vi "nanocal -- nuclear schottky fit V7.vi"() -> ()   [LabVIEW 2021] (continued)
 0.022752418474   ,  \"T\" -> 1.130000000000   ,  \"B\" -> 12.000000000000   ,  \"θ\" -> 45.000000000000   ,  \"Reoff\" -> 0.000000000000   ,  \"Imoff\" -> 0.000000000000   ,  \"στ1\" -> 0.000000000000   ,  \"στS\" -> 0.000000000000   ,  \"στN\" -> 0.000000000000    |>   , \r\"IDS0322_210901_RAW_cal__ref_\" ->   <|    \"ζ\" -> 0.019557893298   ,  \"τ1\" -> 0.012446212333   ,  \"τS\" -> 0.011139553358   ,  \"τN\" -> 0.000114229396   ,  \"τC\" -> 0.005115315079   ,  \"κ0\" -> 0.000000013115   ,  \"mm1\" -> 0.000067933462   ,  \"mm2\" -> 0.012117833487   ,  \"mm3\" -> 0.016849643499   ,  \"T\" -> 1.900000000000   ,  \"B\" -> 12.000000000000   ,  \"θ\" -> 45.000000000000   ,  \"Reoff\" -> 0.000000000000   ,  \"Imoff\" -> 0.000000000000   ,  \"στ1\" -> 0.000000000000   ,  \"στS\" -> 0.000000000000   ,  \"στN\" -> 0.000000000000    |>   , \r\"IDS0322_210901_RAW_cal__sam_\" ->   <|    \"ζ\" -> 0.018090572724   ,  \"τ1\" -> 0.013314780956   ,  \"τS\" -> 0.010820835010   ,  \"τN\" -> 0.000265552167   ,  \"τC\" -> 0.005393540417   ,  \"κ0\" -> 0.000000013100   ,  \"mm1\" -> 0.000064590824   ,  \"mm2\" -> 0.012452255889   ,  \"mm3\" -> 0.017478420931   ,  \"T\" -> 1.900000000000   ,  \"B\" -> 12.000000000000   ,  \"θ\" -> 45.000000000000   ,  \"Reoff\" -> 0.000000000000   ,  \"Imoff\" -> 0.000000000000   ,  \"στ1\" -> 0.000000000000   ,  \"στS\" -> 0.000000000000   ,  \"στN\" -> 0.000000000000    |>   , \r\"IDS0323_210901_RAW_cal__ref_\" ->   <|    \"ζ\" -> 0.018290634783   ,  \"τ1\" -> 0.011707989393   ,  \"τS\" -> 0.007391181448   ,  \"τN\" -> 0.000042685582   ,  \"τC\" -> 0.004638632451   ,  \"κ0\" -> 0.000000023525   ,  \"mm1\" -> 0.000051768819   ,  \"mm2\" -> 0.011185443963   ,  \"mm3\" -> 0.012679246238   ,  \"T\" -> 3.100000000000   ,  \"B\" -> 12.000000000000   ,  \"θ\" -> 45.000000000000   ,  \"Reoff\" -> 0.000000000000   ,  \"Imoff\" -> 0.000000000000   ,  \"στ1\" -> 0.000000000000   ,  \"στS\" -> 0.000000000000   ,  \"στN\" -> 0.000000000000    |>   , \r\"IDS0323_210901_RAW_cal__sam_\" ->   <|    \"ζ\" -> 0.019438138135   ,  \"τ1\" -> 0.013521019406   ,  \"τS\" -> 0.007253169401   ,  \"τN\" -> 0.000154824830   ,  \"τC\" -> 0.004746579385   ,  \"κ0\" -> 0.000000023466   ,  \"mm1\" -> 0.000055371802   ,  \"mm2\" -> 0.011289401344   ,  \"mm3\" -> 0.014474817491   ,  \"T\" -> 3.100000000000   ,  \"B\" -> 12.000000000000   ,  \"θ\" -> 45.000000000000   ,  \"Reoff\" -> 0.000000000000   ,  \"Imoff\" -> 0.000000000000   ,  \"στ1\" -> 0.000000000000   ,  \"στS\" -> 0.000000000000   ,  \"στN\" -> 0.000000000000    |>   , \r\"IDS0324_210901_RAW_cal__ref_\" ->   <|    \"ζ\" -> 0.016342153608   ,  \"τ1\" -> 0.012470308436   ,  \"τS\" -> 0.004793459347   ,  \"τN\" -> 0.000012881713   ,  \"τC\" -> 0.003213848745   ,  \"κ0\" -> 0.000000058321   ,  \"mm1\" -> 0.000031257206   ,  \"mm2\" -> 0.008030763960   ,  \"mm3\" -> 0.012507023039   ,  \"T\" -> 5.700000000000   ,  \"B\" -> 12.000000000000   ,  \"θ\" -> 45.000000000000   ,  \"Reoff\" -> 0.000000000000   ,  \"Imoff\" -> 0.000000000000   ,  \"στ1\" -> 0.000000000000   ,  \"στS\" -> 0.000000000000   ,  \"στN\" -> 0.000000000000    |>   , \r\"IDS0324_210901_RAW_cal__sam_\" ->   <|    \"ζ\" -> 0.018573189054   ,  \"τ1\" -> 0.013304612245   ,  \"τS\" -> 0.003723860844   ,  \"τN\" -> 0.000084829442   ,  \"τC\" -> 0.004309703632   ,  \"κ0\" -> 0.000000058362   ,  \"mm1\" -> 0.000036954445   ,  \"mm2\" -> 0.007938616076   ,  \"mm3\" -> 0.013518175167   ,  \"T\" -> 5.700000000000   ,  \"B\" -> 12.000000000000   ,  \"θ\" -> 45.000000000000   ,  \"Reoff\" -> 0.000000000000   ,  \"Imoff\" -> 0.000000000000   ,  \"στ1\" -> 0.000000000000   ,  \"στS\" -> 0.000000000000   ,  \"στN\" -> 0.000000000000    |>   , \r\"IDS0330_210901_RAW_cal__ref_\" ->   <|    \"ζ\" -> 0.000000000000   ,  \"τ1\" -> 0.000000000000   ,  \"τS\" -> 0.000000000000   ,  \"τN\" -> 0.000000000000   ,  \"τC\" -> 0.000000000000   ,  \"κ0\" -> 0.000000000000   ,  \"mm1\" -> 0.000000000000   ,  \"mm2\" -> 0.000000000000   ,  \"mm3\" -> 0.000000000000   ,  \"T\" -> 0.197000000000   ,  \"B\" -> 1.000000000000   ,  \"θ\" -> 90.000000000000   ,  \"Reoff\" -> 0.000000000000   ,  \"Imoff\" -> 0.000000000000   ,  \"στ1\" -> 0.000000000000   ,  \"στS\" -> 0.000000000000   ,  \"στN\" -> 0.000000000000    |>   , \r\"IDS0330_210901_RAW_cal__sam_\" ->   <|    \"ζ\" -> 0.000000000000   ,  \"τ1\" -> 0.000000000000   ,  \"τS\" -> 0.000000000000   ,  \"τN\" -> 0.000000000000   ,  \"τC\" -> 0.000000000000   ,  \"κ0\" -> 0.000000000000   ,  \"mm1\" -> 0.000000000000   ,  \"mm2\" -> 0.000000000000   ,  \"mm3\" -> 0.000000000000   ,  \"T\" -> 0.197000000000   ,  \"B\" -> 1.000000000000   ,  \"θ\" -> 90.000000000000   ,  \"Reoff\" -> 0.000000000000   ,  \"Imoff\" -> 0.000000000000   ,  \"στ1\" -> 0.000000000000   ,  \"στS\" -> 0.000000000000   ,  \"στN\" -> 0.000000000000    |>   , \r\"IDS0331_210901_RAW_cal__ref_\" ->   <|    \"ζ\" -> 0.000000000000   ,  \"τ1\" -> 0.000000000000   ,  \"τS\" -> 0.000000000000   ,  \"τN\" -> 0.000000000000   ,  \"τC\" -> 0.000000000000   ,  \"κ0\" -> 0.000000000000   ,  \"mm1\" -> 0.000000000000   ,  \"mm2\" -> 0.000000000000   ,  \"mm3\" -> 0.000000000000   ,  \"T\" -> 0.197000000000   ,  \"B\" -> 2.000000000000   ,  \"θ\" -> 90.000000000000   ,  \"Reoff\" -> 0.000000000000   ,  \"Imoff\" -> 0.000000000000   ,  \"στ1\" -> 0.000000000000   ,  \"στS\" -> 0.000000000000   ,  \"στN\" -> 0.000000000000    |>   , \r\"IDS0331_210901_RAW_cal__sam_\" ->   <|    \"ζ\" -> 0.000000000000   ,  \"τ1\" -> 0.000000000000   ,  \"τS\" -> 0.000000000000   ,  \"τN\" -> 0.000000000000   ,  \"τC\" -> 0.000000000000   ,  \"κ0\" -> 0.000000000000   ,  \"mm1\" -> 0.000000000000   ,  \"mm2\" -> 0.000000000000   ,  \"mm3\" -> 0.000000000000   ,  \"T\" -> 0.197000000000   ,  \"B\" -> 2.000000000000   ,  \"θ\" -> 90.000000000000   ,  \"Reoff\" -> 0.000000000000   ,  \"Imoff\" -> 0.000000000000   ,  \"στ1\" -> 0.000000000000   ,  \"στS\" -> 0.000000000000   ,  \"στN\" -> 0.000000000000    |>   , \r\"IDS0335_210904_RAW_cal__ref_\" ->   <|    \"ζ\" -> 0.206204028371   ,  \"τ1\" -> 0.030267809159   ,  \"τS\" -> 0.083699658284   ,  \"τN\" -> 0.011315524001   ,  \"τC\" -> 0.001118356963   ,  \"κ0\" -> 0.000000001029   ,  \"mm1\" -> 0.000189441796   ,  \"mm2\" -> 0.025670987536   ,  \"mm3\" -> 0.120133432419   ,  \"T\" -> 0.197000000000   ,  \"B\" -> 5.000000000000   ,  \"θ\" -> 90.000000000000   ,  \"Reoff\" -> -27794554.455445542900   ,  \"Imoff\" -> 0.000000000000   ,  \"στ1\" -> 0.030199688034   ,  \"στS\" -> 0.003526382549   ,  \"στN\" -> 0.000000000000    |>   , \r\"IDS0335_210904_RAW_cal__sam_\" ->   <|    \"ζ\" -> 0.127476550533   ,  \"τ1\" -> 0.026692349363   ,  \"τS\" -> 0.111739634553   ,  \"τN\" -> 0.012149249884   ,  \"τC\" -> 0.001469649387   ,  \"κ0\" -> 0.000000001130   ,  \"mm1\" -> 0.000164458900   ,  \"mm2\" -> 0.023578369229   ,  \"mm3\" -> 0.144100982695   ,  \"T\" -> 0.197000000000   ,  \"B\" -> 5.000000000000   ,  \"θ\" -> 90.000000000000   ,  \"Reoff\" -> -19117469.879518091700   ,  \"Imoff\" -> 0.000000000000   ,  \"στ1\" -> 0.000000000000   ,  \"στS\" -> 0.000000000000   ,  \"στN\" -> 0.000000000000    |>   , \r\"IDS0336_210904_RAW_cal__ref_\" ->   <|    \"ζ\" -> 0.369061948092   ,  \"τ1\" -> 0.041711176697   ,  \"τS\" -> 0.225950048302   ,  \"τN\" -> 0.066003099748   ,  \"τC\" -> 0.001407606072   ,  \"κ0\" -> 0.000000000381   ,  \"mm1\" -> 0.000378190489   ,  \"mm2\" -> 0.031503380077   ,  \"mm3\" -> 0.410939157824   ,  \"T\" -> 0.122000000000   ,  \"B\" -> 5.000000000000   ,  \"θ\" -> 90.000000000000   ,  \"Reoff\" -> -46126237.623762376600   ,  \"Imoff\" -> 0.000000000000   ,  \"στ1\" -> 0.041981174011   ,  \"στS\" -> 0.019738908124   ,  \"στN\" -> 0.000000000000    |>   , \r\"IDS0336_210904_RAW_cal__sam_\" ->   <|    \"ζ\" -> 0.192483765517   ,  \"τ1\" -> 0.038218926206   ,  \"τS\" -> 0.302700165376   ,  \"τN\" -> 0.092288910100   ,  \"τC\" -> 0.001788727736   ,  \"κ0\" -> 0.000000000500   ,  \"mm1\" -> 0.000287527431   ,  \"mm2\" -> 0.028741269140   ,  \"mm3\" -> 0.481996917433   ,  \"T\" -> 0.122000000000   ,  \"B\" -> 5.000000000000   ,  \"θ\" -> 90.000000000000   ,  \"Reoff\" -> 0.000000000000   ,  \"Imoff\" -> 0.000000000000   ,  \"στ1\" -> 0.000000000000   ,  \"στS\" -> 0.000000000000   ,  \"στN\" -> 0.000000000000    |>   , \r\"IDS0337_210904_RAW_cal__ref_\" ->   <|    \"ζ\" -> 0.291494561804   ,  \"τ1\" -> 0.036667876547   ,  \"τS\" -> 0.128215599927   ,  \"τN\" -> 0.021540574973   ,  \"τC\" -> 0.001127155281   ,  \"κ0\" -> 0.000000000640   ,  \"mm1\" -> 0.000253065243   ,  \"mm2\" -> 0.030442060863   ,  \"mm3\" -> 0.200509191202   ,  \"T\" -> 0.157000000000   ,  \"B\" -> 5.000000000000   ,  \"θ\" -> 90.000000000000   ,  \"Reoff\" -> -62465346.534653462500   ,  \"Imoff\" -> 0.000000000000   ,  \"στ1\" -> 0.039211636627   ,  \"στS\" -> 0.006414125500   ,  \"στN\" -> 0.000000000000    |>   , \r\"IDS0337_210904_RAW_cal__sam_\" ->   <|    \"ζ\" -> 0.174989526301   ,  \"τ1\" -> 0.032277116931   ,  \"τS\" -> 0.156061636315   ,  \"τN\" -> 0.033861256896   ,  \"τC\" -> 0.001461638306   ,  \"κ0\" -> 0.000000000742   ,  \"mm1\" -> 0.000216209109   ,  \"mm2\" -> 0.025810900049   ,  \"mm3\" -> 0.230869056407   ,  \"T\" -> 0.157000000000   ,  \"B\" -> 5.000000000000   ,  \"θ\" -> 90.000000000000   ,  \"Reoff\" -> -41753012.048192769300   ,  \"Imoff\" -> 0.000000000000   ,  \"στ1\" -> 0.000000000000   ,  \"στS\" -> 0.000000000000   ,  \"στN\" -> 0.000000000000    |>   , \r\"IDS0338_210904_RAW_cal__ref_\" ->   <|    \"ζ\" -> 0.269633076560   ,  \"τ1\" -> 0.032794135380   ,  \"τS\" -> 0.108453011647   ,  \"τN\" -> 0.017260666597   ,  \"τC\" -> 0.001066919164   ,  \"κ0\" -> 0.000000000733   ,  \"mm1\" -> 0.000225204386   ,  \"mm2\" -> 0.027393186252   ,  \"mm3\" -> 0.165852907980   ,  \"T\" -> 0.170000000000   ,  \"B\" -> 5.000000000000   ,  \"θ\" -> 90.000000000000   ,  \"Reoff\" -> -53299504.950495049400   ,  \"Imoff\" -> 0.000000000000   ,  \"στ1\" -> 0.032867428442   ,  \"στS\" -> 0.004982833917   ,  \"στN\" -> 0.000000000000    |>   , \r\"IDS0338_210904_RAW_cal__sam_\" ->   <|    \"ζ\" -> 0.165649151389   ,  \"τ1\" -> 0.028874600848   ,  \"τS\" -> 0.141983523605   ,  \"τN\" -> 0.021766467668   ,  \"τC\" -> 0.001383503895   ,  \"κ0\" -> 0.000000000838   ,  \"mm1\" -> 0.000195205233   ,  \"mm2\" -> 0.024502619119   ,  \"mm3\" -> 0.196435318758   ,  \"T\" -> 0.170000000000   ,  \"B\" -> 5.000000000000   ,  \"θ\" -> 90.000000000000   ,  \"Reoff\" -> -35397590.361445784600   ,  \"Imoff\" -> 0.000000000000   ,  \"στ1\" -> 0.000000000000   ,  \"στS\" -> 0.000000000000   ,  \"στN\" -> 0.000000000000    |>   , \r\"IDS0339_210904_RAW_cal__ref_\" ->   <|    \"ζ\" -> 0.118223949911   ,  \"τ1\" -> 0.026953810816   ,  \"τS\" -> 0.059687464570   ,  \"τN\" -> 0.005813068847   ,  \"τC\" -> 0.001318135171   ,  \"κ0\" -> 0.000000001341   ,  \"mm1\" -> 0.000136934905   ,  \"mm2\" -> 0.023512775569   ,  \"mm3\" -> 0.077866500712   ,  \"T\" -> 0.255000000000   ,  \"B\" -> 5.000000000000   ,  \"θ\" -> 90.000000000000   ,  \"Reoff\" -> -14245049.504950493600   ,  \"Imoff\" -> 0.000000000000   ,  \"στ1\" -> 0.036632926849   ,  \"στS\" -> 0.002605706336   ,  \"στN\" -> 0.000000000000    |>   , \r\"IDS0339_210904_RAW_cal__sam_\" ->   <|    \"ζ\" -> 0.070510248751   ,  \"τ1\" -> 0.022152847239   ,  \"τS\" -> 0.078660981887   ,  \"τN\" -> 0.006346817462   ,  \"τC\" -> 0.001852903257   ,  \"κ0\" -> 0.000000001477   ,  \"mm1\" -> 0.000119580835   ,  \"mm2\" -> 0.020081415868   ,  \"mm3\" -> 0.094806474219   ,  \"T\" -> 0.255000000000   ,  \"B\" -> 5.000000000000   ,  \"θ\" -> 90.000000000000   ,  \"Reoff\" -> -9000000.000000000000   ,  \"Imoff\" -> 0.000000000000   ,  \"στ1\" -> 0.000000000000   ,  \"στS\" -> 0.000000000000   ,  \"στN\" -> 0.000000000000    |>   , \r\"IDS0340_210904_RAW_cal__ref_\" ->   <|    \"ζ\" -> 0.082410022210   ,  \"τ1\" -> 0.025302969896   ,  \"τS\" -> 0.049616733190   ,  \"τN\" -> 0.002823484973   ,  \"τC\" -> 0.001541432070   ,  \"κ0\" -> 0.000000001718   ,  \"mm1\" -> 0.000114319399   ,  \"mm2\" -> 0.023099438171   ,  \"mm3\" -> 0.060392462102   ,  \"T\" -> 0.308000000000   ,  \"B\" -> 5.000000000000   ,  \"θ\" -> 90.000000000000   ,  \"Reoff\" -> -7868811.881188109520   ,  \"Imoff\" -> 0.000000000000   ,  \"στ1\" -> 0.036552733909   ,  \"στS\" -> 0.001615668069   ,  \"στN\" -> 0.000000000000    |>   , \r\"IDS0340_210904_RAW_cal__sam_\" ->   <|    \"ζ\" -> 0.049192434897   ,  \"τ1\" -> 0.021139048522   ,  \"τS\" -> 0.064524263818   ,  \"τN\" -> 0.003413094239   ,  \"τC\" -> 0.002227810965   ,  \"κ0\" -> 0.000000001879   ,  \"mm1\" -> 0.000101271202   ,  \"mm2\" -> 0.019728994700   ,  \"mm3\" -> 0.074815955705   ,  \"T\" -> 0.308000000000   ,  \"B\" -> 5.000000000000   ,  \"θ\" -> 90.000000000000   ,  \"Reoff\" -> -4933734.939759036530   ,  \"Imoff\" -> 0.000000000000   ,  \"στ1\" -> 0.000000000000   ,  \"στS\" -> 0.000000000000   ,  \"στN\" -> 0.000000000000    |>   , \r\"IDS0341_210904_RAW_cal__ref_\" ->   <|    \"ζ\" -> 0.059535652055   ,  \"τ1\" -> 0.024399428177   ,  \"τS\" -> 0.042628676419   ,  \"τN\" -> 0.001866665396   ,  \"τC\" -> 0.001976492813   ,  \"κ0\" -> 0.000000002092   ,  \"mm1\" -> 0.000106643977   ,  \"mm2\" -> 0.022574580065   ,  \"mm3\" -> 0.050839097951   ,  \"T\" -> 0.360000000000   ,  \"B\" -> 5.000000000000   ,  \"θ\" -> 90.000000000000   ,  \"Reoff\" -> -3485148.514851480720   ,  \"Imoff\" -> 0.000000000000   ,  \"στ1\" -> 0.049517186258   ,  \"στS\" -> 0.001491570893   ,  \"στN\" -> 0.000000000000    |>   , \r\"IDS0341_210904_RAW_cal__sam_\" ->   <|    \"ζ\" -> 0.036062522071   ,  \"τ1\" -> 0.018116162768   ,  \"τS\" -> 0.055032833309   ,  \"τN\" -> 0.002026723445   ,  \"τC\" -> 0.002755523522   ,  \"κ0\" -> 0.000000002282   ,  \"mm1\" -> 0.000091630452   ,  \"mm2\" -> 0.017261892165   ,  \"mm3\" -> 0.062635431951   ,  \"T\" -> 0.360000000000   ,  \"B\" -> 5.000000000000   ,  \"θ\" -> 90.000000000000   ,  \"Reoff\" -> -2587349.397590361540   ,  \"Imoff\" -> 0.000000000000   ,  \"στ1\" -> 0.000000000000   ,  \"στS\" -> 0.000000000000   ,  \"στN\" -> 0.000000000000    |>   , \r\"IDS0342_210904_RAW_cal__ref_\" ->   <|    \"ζ\" -> 0.044694741546   ,  \"τ1\" -> 0.020073823055   ,  \"τS\" -> 0.035925122531   ,  \"τN\" -> 0.001180968193   ,  \"τC\" -> 0.002238294537   ,  \"κ0\" -> 0.000000002627   ,  \"mm1\" -> 0.000090575996   ,  \"mm2\" -> 0.018946622284   ,  \"mm3\" -> 0.042039457171   ,  \"T\" -> 0.438000000000   ,  \"B\" -> 5.000000000000   ,  \"θ\" -> 90.000000000000   ,  \"Reoff\" -> -2688118.811881184580   ,  \"Imoff\" -> 0.000000000000   ,  \"στ1\" -> 0.000000000000   ,  \"στS\" -> 0.000039598396   ,  \"στN\" -> 0.000000000000    |>   , \r\"IDS0342_210904_RAW_cal__sam_\" ->   <|    \"ζ\" -> 0.027534849374   ,  \"τ1\" -> 0.019066527741   ,  \"τS\" -> 0.046236587360   ,  \"τN\" -> 0.001227722560   ,  \"τC\" -> 0.003332461518   ,  \"κ0\" -> 0.000000002852   ,  \"mm1\" -> 0.000083583563   ,  \"mm2\" -> 0.018352322518   ,  \"mm3\" -> 0.052734315722   ,  \"T\" -> 0.438000000000   ,  \"B\" -> 5.000000000000   ,  \"θ\" -> 90.000000000000   ,  \"Reoff\" -> -1846385.542168676850   ,  \"Imoff\" -> 0.000000000000   ,  \"στ1\" -> 0.000000000000   ,  \"στS\" -> 0.000000000000   ,  \"στN\" -> 0.000000000000    |>   , \r\"IDS0343_210904_RAW_cal__ref_\" ->   <|    \"ζ\" -> 0.035816355504   ,  \"τ1\" -> 0.018852618665   ,  \"τS\" -> 0.030539930714   ,  \"τN\" -> 0.000576682499   ,  \"τC\" -> 0.002754969701   ,  \"κ0\" -> 0.000000003271   ,  \"mm1\" -> 0.000087853298   ,  \"mm2\" -> 0.018179313354   ,  \"mm3\" -> 0.035571518608   ,  \"T\" -> 0.530000000000   ,  \"B\" -> 5.000000000000   ,  \"θ\" -> 90.000000000000   ,  \"Reoff\" -> -1891089.108910888430   ,  \"Imoff\" -> 0.000000000000   ,  \"στ1\" -> 0.000000000000   ,  \"στS\" -> 0.000000000000   ,  \"στN\" -> 0.000000000000    |>   , \r\"IDS0343_210904_RAW_cal__sam_\" ->   <|    \"ζ\" -> 0.023098882919   ,  \"τ1\" -> 0.017709986922   ,  \"τS\" -> 0.038881575014   ,  \"τN\" -> 0.000747654909   ,  \"τC\" -> 0.003803962289   ,  \"κ0\" -> 0.000000003538   ,  \"mm1\" -> 0.000078528513   ,  \"mm2\" -> 0.017209583260   ,  \"mm3\" -> 0.044770458303   ,  \"T\" -> 0.530000000000   ,  \"B\" -> 5.000000000000   ,  \"θ\" -> 90.000000000000   ,  \"Reoff\" -> -1599397.590361446140   ,  \"Imoff\" -> 0.000000000000   ,  \"στ1\" -> 0.000000000000   ,  \"στS\" -> 0.000000000000   ,  \"στN\" -> 0.000000000000    |>   , \r\"IDS0344_210904_RAW_cal__ref_\" ->   <|    \"ζ\" -> 0.030262302634   ,  \"τ1\" -> 0.017398280529   ,  \"τS\" -> 0.027078056707   ,  \"τN\" -> 0.000382363637   ,  \"τC\" -> 0.002680781698   ,  \"κ0\" -> 0.000000003878   ,  \"mm1\" -> 0.000072009464   ,  \"mm2\" -> 0.016908620237   ,  \"mm3\" -> 0.031389868421   ,  \"T\" -> 0.620000000000   ,  \"B\" -> 5.000000000000   ,  \"θ\" -> 90.000000000000   ,  \"Reoff\" -> -1891089.108910888430   ,  \"Imoff\" -> 0.000000000000   ,  \"στ1\" -> 0.000000000000   ,  \"στS\" -> 0.000000000000   ,  \"στN\" -> 0.000000000000    |>   , \r\"IDS0344_210904_RAW_cal__sam_\" ->   <|    \"ζ\" -> 0.019239644947   ,  \"τ1\" -> 0.016162010817   ,  \"τS\" -> 0.033688234899   ,  \"τN\" -> 0.000426792406   ,  \"τC\" -> 0.004393456024   ,  \"κ0\" -> 0.000000004224   ,  \"mm1\" -> 0.000073664779   ,  \"mm2\" -> 0.015859557336   ,  \"mm3\" -> 0.039393633044   ,  \"T\" -> 0.620000000000   ,  \"B\" -> 5.000000000000   ,  \"θ\" -> 90.000000000000   ,  \"Reoff\" -> -1105421.686746988450   ,  \"Imoff\" -> 0.000000000000   ,  \"στ1\" -> 0.000000000000   ,  \"στS\" -> 0.000000000000   ,  \"στN\" -> 0.000000000000    |>   , \r\"IDS0346_210904_RAW_cal__ref_\" ->   <|    \"ζ\" -> 0.358342122070   ,  \"τ1\" -> 0.051761802826   ,  \"τS\" -> 0.089859508524   ,  \"τN\" -> 0.270637714066   ,  \"τC\" -> 0.001160576368   ,  \"κ0\" -> 0.000000000399   ,  \"mm1\" -> 0.000303997839   ,  \"mm2\" -> 0.011999269265   ,  \"mm3\" -> 0.530297674424   ,  \"T\" -> 0.122000000000   ,  \"B\" -> 8.000000000000   ,  \"θ\" -> 90.000000000000   ,  \"Reoff\" -> -78405940.594059407700   ,  \"Imoff\" -> 0.000000000000   ,  \"στ1\" -> 0.018696549634   ,  \"στS\" -> 0.010329197801   ,  \"στN\" -> 0.000000000000    |>   , \r\"IDS0346_210904_RAW_cal__sam_\" ->   <|    \"ζ\" -> 0.199267253863   ,  \"τ1\" -> 0.050205114691   ,  \"τS\" -> 0.125855812683   ,  \"τN\" -> 0.296749666016   ,  \"τC\" -> 0.001624351903   ,  \"κ0\" -> 0.000000000535   ,  \"mm1\" -> 0.000267463038   ,  \"mm2\" -> 0.014047868056   ,  \"mm3\" -> 0.544331047407   ,  \"T\" -> 0.122000000000   ,  \"B\" -> 8.000000000000   ,  \"θ\" -> 90.000000000000   ,  \"Reoff\" -> -35716867.469879508000   ,  \"Imoff\" -> 0.000000000000   ,  \"στ1\" -> 0.000000000000   ,  \"στS\" -> 0.000000000000   ,  \"στN\" -> 0.000000000000    |>   , \r\"IDS0347_210906_RAW_cal__ref_\" ->   <|    \"ζ\" -> 0.284128861979   ,  \"τ1\" -> 0.040855237949   ,  \"τS\" -> 0.067239160062   ,  \"τN\" -> 0.100640688459   ,  \"τC\" -> 0.001094387721   ,  \"κ0\" -> 0.000000000641   ,  \"mm1\" -> 0.000239752131   ,  \"mm2\" -> 0.014685784170   ,  \"mm3\" -> 0.242603448199   ,  \"T\" -> 0.157000000000   ,  \"B\" -> 8.000000000000   ,  \"θ\" -> 90.000000000000   ,  \"Reoff\" -> -67247524.752475246800   ,  \"Imoff\" -> 0.000000000000   ,  \"στ1\" -> 0.009528946219   ,  \"στS\" -> 0.006641775518   ,  \"στN\" -> 0.000000000000    |>   , \r\"IDS0347_210906_RAW_cal__sam_\" ->   <|    \"ζ\" -> 0.169709128246   ,  \"τ1\" -> 0.042569783210   ,  \"τS\" -> 0.096466158196   ,  \"τN\" -> 0.116379310482   ,  \"τC\" -> 0.001498996005   ,  \"κ0\" -> 0.000000000766   ,  \"mm1\" -> 0.000215022431   ,  \"mm2\" -> 0.017656553883   ,  \"mm3\" -> 0.275164490520   ,  \"T\" -> 0.157000000000   ,  \"B\" -> 8.000000000000   ,  \"θ\" -> 90.000000000000   ,  \"Reoff\" -> -35716867.469879508000   ,  \"Imoff\" -> 0.000000000000   ,  \"στ1\" -> 0.000000000000   ,  \"στS\" -> 0.000000000000   ,  \"στN\" -> 0.000000000000    |>   , \r\"IDS0348_210906_RAW_cal__ref_\" ->   <|    \"ζ\" -> 0.229184446116   ,  \"τ1\" -> 0.036521753559   ,  \"τS\" -> 0.056643116422   ,  \"τN\" -> 0.063013769225   ,  \"τC\" -> 0.001114108457   ,  \"κ0\" -> 0.000000000764   ,  \"mm1\" -> 0.000205034245   ,  \"mm2\" -> 0.015217532140   ,  \"mm3\" -> 0.169293678338   ,  \"T\" -> 0.178000000000   ,  \"B\" -> 8.000000000000   ,  \"θ\" -> 90.000000000000   ,  \"Reoff\" -> -44930693.069306924900   ,  \"Imoff\" -> 0.000000000000   ,  \"στ1\" -> 0.007491304915   ,  \"στS\" -> 0.004191211320   ,  \"στN\" -> 0.000000000000    |>   , \r\"IDS0348_210906_RAW_cal__sam_\" ->   <|    \"ζ\" -> 0.135783247929   ,  \"τ1\" -> 0.037121050091   ,  \"τS\" -> 0.079201640502   ,  \"τN\" -> 0.079201640502   ,  \"τC\" -> 0.001474311209   ,  \"κ0\" -> 0.000000000894   ,  \"mm1\" -> 0.000173730712   ,  \"mm2\" -> 0.016810842330   ,  \"mm3\" -> 0.201522581240   ,  \"T\" -> 0.178000000000   ,  \"B\" -> 8.000000000000   ,  \"θ\" -> 90.000000000000   ,  \"Reoff\" -> -29680722.891566276600   ,  \"Imoff\" -> 0.000000000000   ,  \"στ1\" -> 0.000000000000   ,  \"στS\" -> 0.000000000000   ,  \"στN\" -> 0.000000000000    |>   , \r\"IDS0349_210906_RAW_cal__ref_\" ->   <|    \"ζ\" -> 0.190984000958   ,  \"τ1\" -> 0.032898392235   ,  \"τS\" -> 0.053015075726   ,  \"τN\" -> 0.036446539803   ,  \"τC\" -> 0.001170894868   ,  \"κ0\" -> 0.000000001035   ,  \"mm1\" -> 0.000184864342   ,  \"mm2\" -> 0.017107531018   ,  \"mm3\" -> 0.123324244538   ,  \"T\" -> 0.200000000000   ,  \"B\" -> 8.000000000000   ,  \"θ\" -> 90.000000000000   ,  \"Reoff\" -> -24207920.792079202800   ,  \"Imoff\" -> 0.000000000000   ,  \"στ1\" -> 0.007827965999   ,  \"στS\" -> 0.003040573624   ,  \"στN\" -> 0.000000000000    |>   , \r\"IDS0349_210906_RAW_cal__sam_\" ->   <|    \"ζ\" -> 0.113690190882   ,  \"τ1\" -> 0.032691214581   ,  \"τS\" -> 0.068786957350   ,  \"τN\" -> 0.048058332081   ,  \"τC\" -> 0.001613875480   ,  \"κ0\" -> 0.000000001156   ,  \"mm1\" -> 0.000161675745   ,  \"mm2\" -> 0.017372504664   ,  \"mm3\" -> 0.146900362342   ,  \"T\" -> 0.200000000000   ,  \"B\" -> 8.000000000000   ,  \"θ\" -> 90.000000000000   ,  \"Reoff\" -> -14590361.445783138300   ,  \"Imoff\" -> 0.000000000000   ,  \"στ1\" -> 0.000000000000   ,  \"στS\" -> 0.000000000000   ,  \"στN\" -> 0.000000000000    |>   , \r\"IDS0350_210906_RAW_cal__ref_\" ->   <|    \"ζ\" -> 0.117284187691   ,  \"τ1\" -> 0.026970666142   ,  \"τS\" -> 0.042347096729   ,  \"τN\" -> 0.016129848116   ,  \"τC\" -> 0.001330224146   ,  \"κ0\" -> 0.000000001350   ,  \"mm1\" -> 0.000136193348   ,  \"mm2\" -> 0.017132196816   ,  \"mm3\" -> 0.076367865944   ,  \"T\" -> 0.260000000000   ,  \"B\" -> 8.000000000000   ,  \"θ\" -> 90.000000000000   ,  \"Reoff\" -> -13846534.653465345500   ,  \"Imoff\" -> 0.000000000000   ,  \"στ1\" -> 0.008626446357   ,  \"στS\" -> 0.001916708788   ,  \"στN\" -> 0.000000000000    |>   , \r\"IDS0350_210906_RAW_cal__sam_\" ->   <|    \"ζ\" -> 0.071614468485   ,  \"τ1\" -> 0.024327525692   ,  \"τS\" -> 0.055056024171   ,  \"τN\" -> 0.019709093999   ,  \"τC\" -> 0.001754398678   ,  \"κ0\" -> 0.000000001497   ,  \"mm1\" -> 0.000114067222   ,  \"mm2\" -> 0.016460052715   ,  \"mm3\" -> 0.089627186802   ,  \"T\" -> 0.260000000000   ,  \"B\" -> 8.000000000000   ,  \"θ\" -> 90.000000000000   ,  \"Reoff\" -> -10063253.012048184900   ,  \"Imoff\" -> 0.000000000000   ,  \"στ1\" -> 0.000000000000   ,  \"στS\" -> 0.000000000000   ,  \"στN\" -> 0.000000000000    |>   , \r\"IDS0351_210906_RAW_cal__ref_\" ->   <|    \"ζ\" -> 0.080944960576   ,  \"τ1\" -> 0.020924370017   ,  \"τS\" -> 0.037011167707   ,  \"τN\" -> 0.007898683051   ,  \"τC\" -> 0.001560823327   ,  \"κ0\" -> 0.000000001762   ,  \"mm1\" -> 0.000112792747   ,  \"mm2\" -> 0.015713715797   ,  \"mm3\" -> 0.055203761657   ,  \"T\" -> 0.310000000000   ,  \"B\" -> 8.000000000000   ,  \"θ\" -> 90.000000000000   ,  \"Reoff\" -> -7470297.029702961450   ,  \"Imoff\" -> 0.000000000000   ,  \"στ1\" -> 0.010612052509   ,  \"στS\" -> 0.001485327080   ,  \"στN\" -> 0.000000000000    |>   , \r\"IDS0351_210906_RAW_cal__sam_\" ->   <|    \"ζ\" -> 0.049866383839   ,  \"τ1\" -> 0.023285662985   ,  \"τS\" -> 0.049370833464   ,  \"τN\" -> 0.009866658615   ,  \"τC\" -> 0.002153040267   ,  \"κ0\" -> 0.000000001928   ,  \"mm1\" -> 0.000098362318   ,  \"mm2\" -> 0.018063601956   ,  \"mm3\" -> 0.069468190575   ,  \"T\" -> 0.310000000000   ,  \"B\" -> 8.000000000000   ,  \"θ\" -> 90.000000000000   ,  \"Reoff\" -> -5536144.578313261270   ,  \"Imoff\" -> 0.000000000000   ,  \"στ1\" -> 0.000000000000   ,  \"στS\" -> 0.000000000000   ,  \"στN\" -> 0.000000000000    |>   , \r\"IDS0352_210906_RAW_cal__ref_\" ->   <|    \"ζ\" -> 0.059924344954   ,  \"τ1\" -> 0.020444284414   ,  \"τS\" -> 0.034342319161   ,  \"τN\" -> 0.004837568639   ,  \"τC\" -> 0.001951892428   ,  \"κ0\" -> 0.000000002109   ,  \"mm1\" -> 0.000105020639   ,  \"mm2\" -> 0.016539029426   ,  \"mm3\" -> 0.047279843688   ,  \"T\" -> 0.360000000000   ,  \"B\" -> 8.000000000000   ,  \"θ\" -> 90.000000000000   ,  \"Reoff\" -> -3485148.514851480720   ,  \"Imoff\" -> 0.000000000000   ,  \"στ1\" -> 0.016824807524   ,  \"στS\" -> 0.001463681226   ,  \"στN\" -> 0.000000000000    |>   , \r\"IDS0352_210906_RAW_cal__sam_\" ->   <|    \"ζ\" -> 0.036116393265   ,  \"τ1\" -> 0.020310974732   ,  \"τS\" -> 0.044594628397   ,  \"τN\" -> 0.005932938101   ,  \"τC\" -> 0.002747123875   ,  \"κ0\" -> 0.000000002292   ,  \"mm1\" -> 0.000090548575   ,  \"mm2\" -> 0.017024776182   ,  \"mm3\" -> 0.058295213810   ,  \"T\" -> 0.360000000000   ,  \"B\" -> 8.000000000000   ,  \"θ\" -> 90.000000000000   ,  \"Reoff\" -> -2518072.289156645540   ,  \"Imoff\" -> 0.000000000000   ,  \"στ1\" -> 0.000000000000   ,  \"στS\" -> 0.000000000000   ,  \"στN\" -> 0.000000000000    |>   , \r\"IDS0353_210906_RAW_cal__ref_\" ->   <|    \"ζ\" -> 0.045101316453   ,  \"τ1\" -> 0.020505895958   ,  \"τS\" -> 0.031209032196   ,  \"τN\" -> 0.002683750708   ,  \"τC\" -> 0.002226651105   ,  \"κ0\" -> 0.000000002626   ,  \"mm1\" -> 0.000090181690   ,  \"mm2\" -> 0.017621773769   ,  \"mm3\" -> 0.040441983634   ,  \"T\" -> 0.438000000000   ,  \"B\" -> 8.000000000000   ,  \"θ\" -> 90.000000000000   ,  \"Reoff\" -> -2688118.811881184580   ,  \"Imoff\" -> 0.000000000000   ,  \"στ1\" -> 0.000000000000   ,  \"στS\" -> 0.000000000000   ,  \"στN\" -> 0.000000000000    |>   , \r\"IDS0353_210906_RAW_cal__sam_\" ->   <|    \"ζ\" -> 0.028235631162   ,  \"τ1\" -> 0.018033623612   ,  \"τS\" -> 0.040112967891   ,  \"τN\" -> 0.003332308168   ,  \"τC\" -> 0.002994357278   ,  \"κ0\" -> 0.000000002859   ,  \"mm1\" -> 0.000076791949   ,  \"mm2\" -> 0.016073609718   ,  \"mm3\" -> 0.049549560072   ,  \"T\" -> 0.438000000000   ,  \"B\" -> 8.000000000000   ,  \"θ\" -> 90.000000000000   ,  \"Reoff\" -> -2200000.000000000000   ,  \"Imoff\" -> 0.000000000000   ,  \"στ1\" -> 0.000000000000   ,  \"στS\" -> 0.000000000000   ,  \"στN\" -> 0.000000000000    |>   , \r\"IDS0354_210906_RAW_cal__ref_\" ->   <|    \"ζ\" -> 0.035449186867   ,  \"τ1\" -> 0.018569718484   ,  \"τS\" -> 0.028160564144   ,  \"τN\" -> 0.001513040869   ,  \"τC\" -> 0.002627412191   ,  \"κ0\" -> 0.000000003276   ,  \"mm1\" -> 0.000082729429   ,  \"mm2\" -> 0.016803631201   ,  \"mm3\" -> 0.035036280227   ,  \"T\" -> 0.530000000000   ,  \"B\" -> 8.000000000000   ,  \"θ\" -> 90.000000000000   ,  \"Reoff\" -> -2000000.000000000000   ,  \"Imoff\" -> 0.000000000000   ,  \"στ1\" -> 0.000000000000   ,  \"στS\" -> 0.000000000000   ,  \"στN\" -> 0.000000000000    |>   , \r\"IDS0354_210906_RAW_cal__sam_\" ->   <|    \"ζ\" -> 0.022962333090   ,  \"τ1\" -> 0.020865157142   ,  \"τS\" -> 0.035948400917   ,  \"τN\" -> 0.001990138096   ,  \"τC\" -> 0.003574397791   ,  \"κ0\" -> 0.000000003542   ,  \"mm1\" -> 0.000073258085   ,  \"mm2\" -> 0.019040364220   ,  \"mm3\" -> 0.044135629011   ,  \"T\" -> 0.530000000000   ,  \"B\" -> 8.000000000000   ,  \"θ\" -> 90.000000000000   ,  \"Reoff\" -> -1700000.000000000000   ,  \"Imoff\" -> 0.000000000000   ,  \"στ1\" -> 0.000000000000   ,  \"στS\" -> 0.000000000000   ,  \"στN\" -> 0.000000000000    |>   , \r\"IDS0355_210906_RAW_cal__ref_\" ->   <|    \"ζ\" -> 0.023121987816   ,  \"τ1\" -> 0.018681929200   ,  \"τS\" -> 0.017398280529   ,  \"τN\" -> 0.000397568997   ,  \"τC\" -> 0.004006240914   ,  \"κ0\" -> 0.000000005416   ,  \"mm1\" -> 0.000074156421   ,  \"mm2\" -> 0.017157833141   ,  \"mm3\" -> 0.023663505495   ,  \"T\" -> 0.830000000000   ,  \"B\" -> 8.000000000000   ,  \"θ\" -> 90.000000000000   ,  \"Reoff\" -> -695544.554455444216   ,  \"Imoff\" -> 0.000000000000   ,  \"στ1\" -> 0.000000000000   ,  \"στS\" -> 0.000000000000   ,  \"στN\" -> 0.000000000000    |>   , \r\"IDS0355_210906_RAW_cal__sam_\" ->   <|    \"ζ\" -> 0.015987398390   ,  \"τ1\" -> 0.023974349678   ,  \"τS\" -> 0.025824294014   ,  \"τN\" -> 0.000573136357   ,  \"τC\" -> 0.005688548480   ,  \"κ0\" -> 0.000000005865   ,  \"mm1\" -> 0.000073733721   ,  \"mm2\" -> 0.022561297233   ,  \"mm3\" -> 0.033847323811   ,  \"T\" -> 0.830000000000   ,  \"B\" -> 8.000000000000   ,  \"θ\" -> 90.000000000000   ,  \"Reoff\" -> -599999.999999999999   ,  \"Imoff\" -> 0.000000000000   ,  \"στ1\" -> 0.000000000000   ,  \"στS\" -> 0.000000000000   ,  \"στN\" -> 0.000000000000    |>   , \r\"IDS0359_210907_RAW_cal__ref_\" ->   <|    \"ζ\" -> 0.381969883498   ,  \"τ1\" -> 0.094329379305   ,  \"τS\" -> 0.076928325275   ,  \"τN\" -> 0.550887477218   ,  \"τC\" -> 0.001034779226   ,  \"κ0\" -> 0.000000000383   ,  \"mm1\" -> 0.000283958299   ,  \"mm2\" -> 0.010609033514   ,  \"mm3\" -> 0.952093698147   ,  \"T\" -> 0.120000000000   ,  \"B\" -> 12.000000000000   ,  \"θ\" -> 60.000000000000   ,  \"Reoff\" -> -100000000.000000000000   ,  \"Imoff\" -> 0.000000000000   ,  \"στ1\" -> 0.012489604376   ,  \"στS\" -> 0.015785658114   ,  \"στN\" -> 0.000000000000    |>   , \r\"IDS0359_210907_RAW_cal__sam_\" ->   <|    \"ζ\" -> 0.241762987309   ,  \"τ1\" -> 0.090301757431   ,  \"τS\" -> 0.104468976957   ,  \"τN\" -> 0.810352557873   ,  \"τC\" -> 0.001702208121   ,  \"κ0\" -> 0.000000000500   ,  \"mm1\" -> 0.000327834342   ,  \"mm2\" -> 0.009723084216   ,  \"mm3\" -> 1.217944568939   ,  \"T\" -> 0.120000000000   ,  \"B\" -> 12.000000000000   ,  \"θ\" -> 60.000000000000   ,  \"Reoff\" -> -52289156.626506023100   ,  \"Imoff\" -> 0.000000000000   ,  \"στ1\" -> 0.000000000000   ,  \"στS\" -> 0.000000000000   ,  \"στN\" -> 0.000000000000    |>   , \r\"IDS0360_210907_RAW_cal__ref_\" ->   <|    \"ζ\" -> 0.332032071502   ,  \"τ1\" -> 0.077785863829   ,  \"τS\" -> 0.054247117088   ,  \"τN\" -> 0.276531096522   ,  \"τC\" -> 0.001063816056   ,  \"κ0\" -> 0.000000000641   ,  \"mm1\" -> 0.000262214679   ,  \"mm2\" -> 0.011189186969   ,  \"mm3\" -> 0.508005467320   ,  \"T\" -> 0.150000000000   ,  \"B\" -> 12.000000000000   ,  \"θ\" -> 60.000000000000   ,  \"Reoff\" -> -64885542.168674700000   ,  \"Imoff\" -> 0.000000000000   ,  \"στ1\" -> 0.010441701195   ,  \"στS\" -> 0.005858449647   ,  \"στN\" -> 0.000000000000    |>   , \r\"IDS0360_210907_RAW_cal__sam_\" ->   <|    \"ζ\" -> 0.201278537585   ,  \"τ1\" -> 0.081544073952   ,  \"τS\" -> 0.088995303529   ,  \"τN\" -> 0.405130496924   ,  \"τC\" -> 0.001460686320   ,  \"κ0\" -> 0.000000000739   ,  \"mm1\" -> 0.000241947199   ,  \"mm2\" -> 0.013299947862   ,  \"mm3\" -> 0.663045584163   ,  \"T\" -> 0.150000000000   ,  \"B\" -> 12.000000000000   ,  \"θ\" -> 60.000000000000   ,  \"Reoff\" -> -39048192.771084338400   ,  \"Imoff\" -> 0.000000000000   ,  \"στ1\" -> 0.000000000000   ,  \"στS\" -> 0.000000000000   ,  \"στN\" -> 0.000000000000    |>   , \r\"IDS0361_210908_RAW_cal__ref_\" ->   <|    \"ζ\" -> 0.279785391024   ,  \"τ1\" -> 0.067061821351   ,  \"τS\" -> 0.048033272534   ,  \"τN\" -> 0.170024512607   ,  \"τC\" -> 0.001016043022   ,  \"κ0\" -> 0.000000000755   ,  \"mm1\" -> 0.000219251026   ,  \"mm2\" -> 0.012488143188   ,  \"mm3\" -> 0.334437637981   ,  \"T\" -> 0.168000000000   ,  \"B\" -> 12.000000000000   ,  \"θ\" -> 60.000000000000   ,  \"Reoff\" -> -50271084.337349399900   ,  \"Imoff\" -> 0.000000000000   ,  \"στ1\" -> 0.007974659835   ,  \"στS\" -> 0.004537587745   ,  \"στN\" -> 0.000000000000    |>   , \r\"IDS0361_210908_RAW_cal__sam_\" ->   <|    \"ζ\" -> 0.166104690940   ,  \"τ1\" -> 0.071049175548   ,  \"τS\" -> 0.068661809155   ,  \"τN\" -> 0.222482953546   ,  \"τC\" -> 0.001364223445   ,  \"κ0\" -> 0.000000000861   ,  \"mm1\" -> 0.000191495940   ,  \"mm2\" -> 0.014533832786   ,  \"mm3\" -> 0.397193343795   ,  \"T\" -> 0.168000000000   ,  \"B\" -> 12.000000000000   ,  \"θ\" -> 60.000000000000   ,  \"Reoff\" -> -34789156.626506023100   ,  \"Imoff\" -> 0.000000000000   ,  \"στ1\" -> 0.000000000000   ,  \"στS\" -> 0.000000000000   ,  \"στN\" -> 0.000000000000    |>   , \r\"IDS0362_210908_RAW_cal__ref_\" ->   <|    \"ζ\" -> 0.207142334401   ,  \"τ1\" -> 0.057894480183   ,  \"τS\" -> 0.038690220204   ,  \"τN\" -> 0.092417014932   ,  \"τC\" -> 0.001098696065   ,  \"κ0\" -> 0.000000001038   ,  \"mm1\" -> 0.000184887893   ,  \"mm2\" -> 0.013547417032   ,  \"mm3\" -> 0.203525965202   ,  \"T\" -> 0.197000000000   ,  \"B\" -> 12.000000000000   ,  \"θ\" -> 60.000000000000   ,  \"Reoff\" -> -28512048.192771077200   ,  \"Imoff\" -> 0.000000000000   ,  \"στ1\" -> 0.006011065509   ,  \"στS\" -> 0.002598249147   ,  \"στN\" -> 0.000000000000    |>   , \r\"IDS0362_210908_RAW_cal__sam_\" ->   <|    \"ζ\" -> 0.123741217510   ,  \"τ1\" -> 0.059103977068   ,  \"τS\" -> 0.051096152058   ,  \"τN\" -> 0.122661863704   ,  \"τC\" -> 0.001502836172   ,  \"κ0\" -> 0.000000001149   ,  \"mm1\" -> 0.000161683871   ,  \"mm2\" -> 0.014394250129   ,  \"mm3\" -> 0.241309923424   ,  \"T\" -> 0.197000000000   ,  \"B\" -> 12.000000000000   ,  \"θ\" -> 60.000000000000   ,  \"Reoff\" -> -17448795.180722892300   ,  \"Imoff\" -> 0.000000000000   ,  \"στ1\" -> 0.000000000000   ,  \"στS\" -> 0.000000000000   ,  \"στN\" -> 0.000000000000    |>   , \r\"IDS0363_210908_RAW_cal__ref_\" ->   <|    \"ζ\" -> 0.123120408408   ,  \"τ1\" -> 0.041426792490   ,  \"τS\" -> 0.030611483740   ,  \"τN\" -> 0.033673862745   ,  \"τC\" -> 0.001247428044   ,  \"κ0\" -> 0.000000001354   ,  \"mm1\" -> 0.000132437169   ,  \"mm2\" -> 0.014700070997   ,  \"mm3\" -> 0.100041896966   ,  \"T\" -> 0.250000000000   ,  \"B\" -> 12.000000000000   ,  \"θ\" -> 60.000000000000   ,  \"Reoff\" -> -14912650.602409631000   ,  \"Imoff\" -> 0.000000000000   ,  \"στ1\" -> 0.005277736765   ,  \"στS\" -> 0.001423482809   ,  \"στN\" -> 0.000000000000    |>   , \r\"IDS0363_210908_RAW_cal__sam_\" ->   <|    \"ζ\" -> 0.074359211271   ,  \"τ1\" -> 0.044477620306   ,  \"τS\" -> 0.040449563551   ,  \"τN\" -> 0.044745540249   ,  \"τC\" -> 0.001712765821   ,  \"κ0\" -> 0.000000001493   ,  \"mm1\" -> 0.000114327803   ,  \"mm2\" -> 0.016556677808   ,  \"mm3\" -> 0.121049525039   ,  \"T\" -> 0.250000000000   ,  \"B\" -> 12.000000000000   ,  \"θ\" -> 60.000000000000   ,  \"Reoff\" -> -10147590.361445784600   ,  \"Imoff\" -> 0.000000000000   ,  \"στ1\" -> 0.000000000000   ,  \"στS\" -> 0.000000000000   ,  \"στN\" -> 0.000000000000    |>   , \r\"IDS0364_210908_RAW_cal__ref_\" ->   <|    \"ζ\" -> 0.083964366121   ,  \"τ1\" -> 0.035864566651   ,  \"τS\" -> 0.027410501881   ,  \"τN\" -> 0.017171198615   ,  \"τC\" -> 0.001554769636   ,  \"κ0\" -> 0.000000001739   ,  \"mm1\" -> 0.000114855748   ,  \"mm2\" -> 0.016061286678   ,  \"mm3\" -> 0.069568168580   ,  \"T\" -> 0.307000000000   ,  \"B\" -> 12.000000000000   ,  \"θ\" -> 60.000000000000   ,  \"Reoff\" -> -7659638.554216861730   ,  \"Imoff\" -> 0.000000000000   ,  \"στ1\" -> 0.006264566865   ,  \"στS\" -> 0.001087528836   ,  \"στN\" -> 0.000000000000    |>   , \r\"IDS0364_210908_RAW_cal__sam_\" ->   <|    \"ζ\" -> 0.051560123380   ,  \"τ1\" -> 0.037167172913   ,  \"τS\" -> 0.035875072163   ,  \"τN\" -> 0.021782945969   ,  \"τC\" -> 0.002191662682   ,  \"κ0\" -> 0.000000001902   ,  \"mm1\" -> 0.000101812126   ,  \"mm2\" -> 0.018093196790   ,  \"mm3\" -> 0.081794699340   ,  \"T\" -> 0.307000000000   ,  \"B\" -> 12.000000000000   ,  \"θ\" -> 60.000000000000   ,  \"Reoff\" -> -5584337.349397592250   ,  \"Imoff\" -> 0.000000000000   ,  \"στ1\" -> 0.000000000000   ,  \"στS\" -> 0.000000000000   ,  \"στN\" -> 0.000000000000    |>   , \r\"IDS0365_210908_RAW_cal__ref_\" ->   <|    \"ζ\" -> 0.061646569706   ,  \"τ1\" -> 0.029620794864   ,  \"τS\" -> 0.025192478366   ,  \"τN\" -> 0.009702290524   ,  \"τC\" -> 0.001914430909   ,  \"κ0\" -> 0.000000002114   ,  \"mm1\" -> 0.000104108758   ,  \"mm2\" -> 0.016173173755   ,  \"mm3\" -> 0.052303854953   ,  \"T\" -> 0.360000000000   ,  \"B\" -> 12.000000000000   ,  \"θ\" -> 60.000000000000   ,  \"Reoff\" -> -4033132.530120491980   ,  \"Imoff\" -> 0.000000000000   ,  \"στ1\" -> 0.007715852130   ,  \"στS\" -> 0.000971919235   ,  \"στN\" -> 0.000000000000    |>   , \r\"IDS0365_210908_RAW_cal__sam_\" ->   <|    \"ζ\" -> 0.037527154631   ,  \"τ1\" -> 0.031791574880   ,  \"τS\" -> 0.032568278603   ,  \"τN\" -> 0.012463984296   ,  \"τC\" -> 0.002682405917   ,  \"κ0\" -> 0.000000002306   ,  \"mm1\" -> 0.000090102201   ,  \"mm2\" -> 0.018466994147   ,  \"mm3\" -> 0.062639080041   ,  \"T\" -> 0.360000000000   ,  \"B\" -> 12.000000000000   ,  \"θ\" -> 60.000000000000   ,  \"Reoff\" -> -2846385.542168676850   ,  \"Imoff\" -> 0.000000000000   ,  \"στ1\" -> 0.000000000000   ,  \"στS\" -> 0.000000000000   ,  \"στN\" -> 0.000000000000    |>   , \r\"IDS0366_210908_RAW_cal__ref_\" ->   <|    \"ζ\" -> 0.045512932741   ,  \"τ1\" -> 0.026001941230   ,  \"τS\" -> 0.023139529347   ,  \"τN\" -> 0.005224117100   ,  \"τC\" -> 0.002327747283   ,  \"κ0\" -> 0.000000002647   ,  \"mm1\" -> 0.000092754843   ,  \"mm2\" -> 0.016672258116   ,  \"mm3\" -> 0.041219234735   ,  \"T\" -> 0.430000000000   ,  \"B\" -> 12.000000000000   ,  \"θ\" -> 60.000000000000   ,  \"Reoff\" -> -2219879.518072277310   ,  \"Imoff\" -> 0.000000000000   ,  \"στ1\" -> 0.011333887810   ,  \"στS\" -> 0.000897031833   ,  \"στN\" -> 0.000000000000    |>   , \r\"IDS0366_210908_RAW_cal__sam_\" ->   <|    \"ζ\" -> 0.029143715364   ,  \"τ1\" -> 0.026198855926   ,  \"τS\" -> 0.029745373312   ,  \"τN\" -> 0.006649011545   ,  \"τC\" -> 0.003090491846   ,  \"κ0\" -> 0.000000002869   ,  \"mm1\" -> 0.000079676072   ,  \"mm2\" -> 0.018163106475   ,  \"mm3\" -> 0.048501617675   ,  \"T\" -> 0.430000000000   ,  \"B\" -> 12.000000000000   ,  \"θ\" -> 60.000000000000   ,  \"Reoff\" -> -2237951.807228915390   ,  \"Imoff\" -> 0.000000000000   ,  \"στ1\" -> 0.000000000000   ,  \"στS\" -> 0.000000000000   ,  \"στN\" -> 0.000000000000    |>   , \r\"IDS0367_210908_RAW_cal__ref_\" ->   <|    \"ζ\" -> 0.037324451442   ,  \"τ1\" -> 0.019605264024   ,  \"τS\" -> 0.021700560504   ,  \"τN\" -> 0.002800944156   ,  \"τC\" -> 0.002526998509   ,  \"κ0\" -> 0.000000003301   ,  \"mm1\" -> 0.000082012466   ,  \"mm2\" -> 0.015132192259   ,  \"mm3\" -> 0.032334067689   ,  \"T\" -> 0.530000000000   ,  \"B\" -> 12.000000000000   ,  \"θ\" -> 60.000000000000   ,  \"Reoff\" -> 0.000000000000   ,  \"Imoff\" -> 0.000000000000   ,  \"στ1\" -> 0.000000000000   ,  \"στS\" -> 0.000000000000   ,  \"στN\" -> 0.000000000000    |>   , \r\"IDS0367_210908_RAW_cal__sam_\" ->   <|    \"ζ\" -> 0.024637271207   ,  \"τ1\" -> 0.025634847148   ,  \"τS\" -> 0.027302474030   ,  \"τN\" -> 0.003538185279   ,  \"τC\" -> 0.003933377133   ,  \"κ0\" -> 0.000000003566   ,  \"mm1\" -> 0.000083131278   ,  \"mm2\" -> 0.019726981228   ,  \"mm3\" -> 0.041358600771   ,  \"T\" -> 0.530000000000   ,  \"B\" -> 12.000000000000   ,  \"θ\" -> 60.000000000000   ,  \"Reoff\" -> -1629518.072289161380   ,  \"Imoff\" -> 0.000000000000   ,  \"στ1\" -> 0.000000000000   ,  \"στS\" -> 0.000000000000   ,  \"στN\" -> 0.000000000000    |>   , \r\"IDS0368_210908_RAW_cal__ref_\" ->   <|    \"ζ\" -> 0.030581023885   ,  \"τ1\" -> 0.017326525290   ,  \"τS\" -> 0.020225378130   ,  \"τN\" -> 0.001703135365   ,  \"τC\" -> 0.003380889395   ,  \"κ0\" -> 0.000000003914   ,  \"mm1\" -> 0.000086626446   ,  \"mm2\" -> 0.014628874360   ,  \"mm3\" -> 0.028591023770   ,  \"T\" -> 0.630000000000   ,  \"B\" -> 12.000000000000   ,  \"θ\" -> 60.000000000000   ,  \"Reoff\" -> 0.000000000000   ,  \"Imoff\" -> 0.000000000000   ,  \"στ1\" -> 0.000000000000   ,  \"στS\" -> 0.000000000000   ,  
